vi "Terminal-PressureSystem-DeviceLubricateUnit-Getter.vi"(8 "error in (no error)":errorcluster caption="错误输入（无错误）", 11 "read operation timeout (ms)":i32=5000 caption="读操作超时（5000毫秒）") -> (0 "error out":errorcluster caption="错误输出", 2 "时间标识":timestamp, 3 "液压子系统陪试润滑单元":T1)   [LabVIEW 2014]
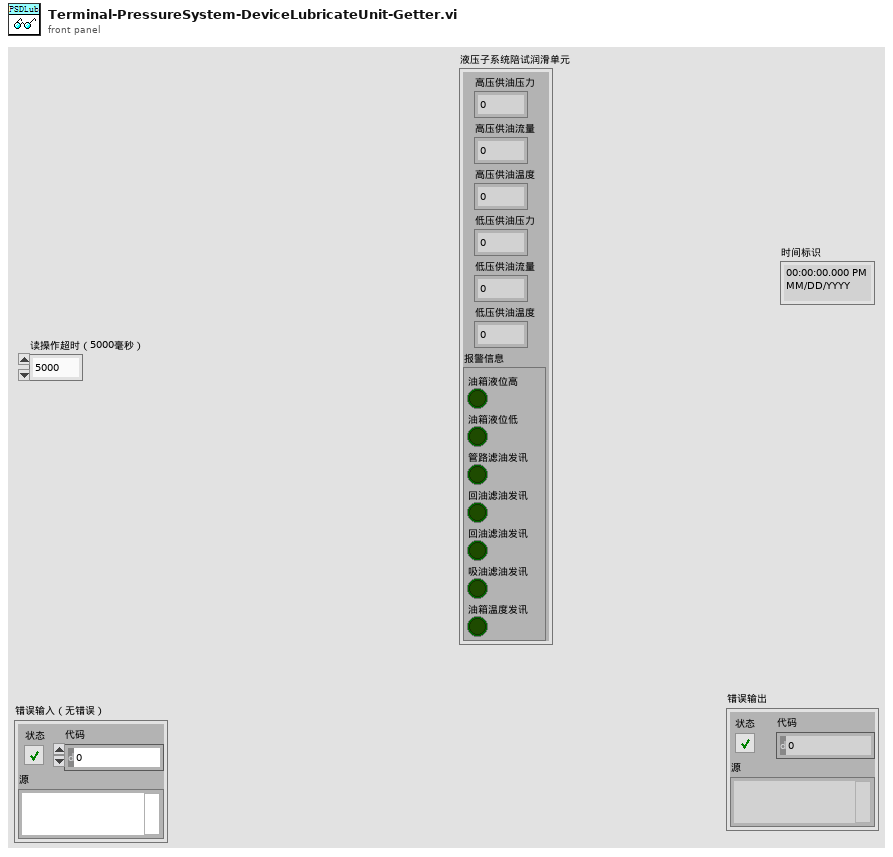
[diagram p1: front panel]
types:
  T1 = cluster{"高压供油压力":u16, "高压供油流量":u16, "高压供油温度":u16, "低压供油压力":u16, "低压供油流量":u16, "低压供油温度":u16, "报警信息":cluster{"油箱液位高":bool, "油箱液位低":bool, "管路滤油发讯":bool, "回油滤油发讯":bool, "回油滤油发讯":bool, "吸油滤油发讯":bool, "油箱温度发讯":bool}}
  T2 = cluster{"油箱液位高":bool, "油箱液位低":bool, "管路滤油发讯":bool, "回油滤油发讯":bool, "回油滤油发讯":bool, "吸油滤油发讯":bool, "油箱温度发讯":bool}
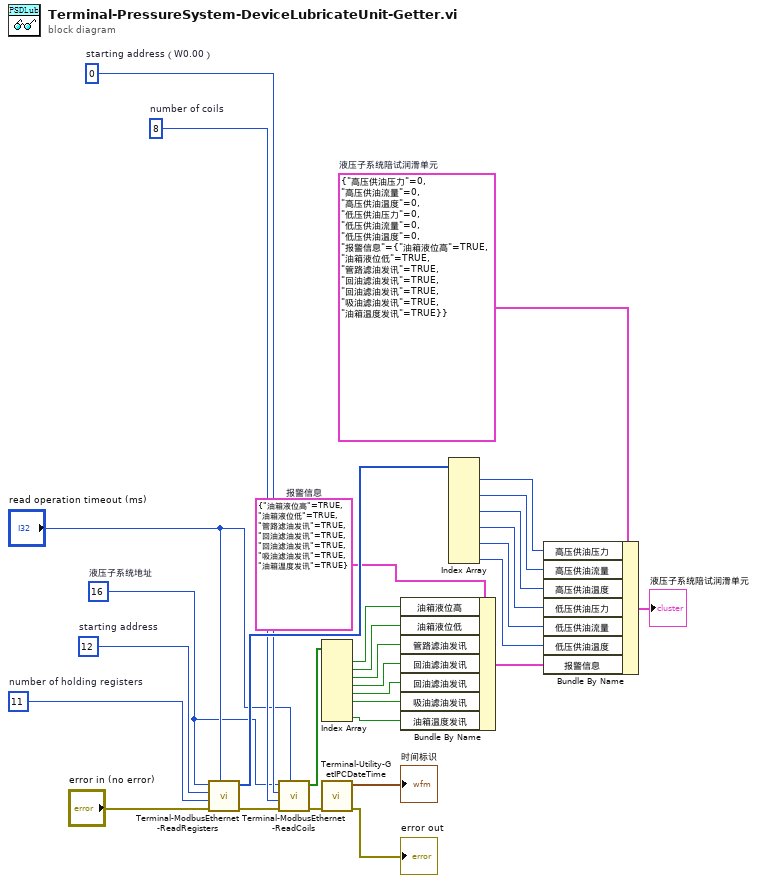
[diagram p0: block diagram]
diagram:
  w12 = T2 {"油箱液位高"=TRUE, "油箱液位低"=TRUE, "管路滤油发讯"=TRUE, "回油滤油发讯"=TRUE, "回油滤油发讯"=TRUE, "吸油滤油发讯"=TRUE, "油箱温度发讯"=TRUE}  # 报警信息
  w21 = u16 8  # number of coils
  w22 = u16 0  # starting address（W0.00）
  w28 = T1 {"高压供油压力"=0, "高压供油流量"=0, "高压供油温度"=0, "低压供油压力"=0, "低压供油流量"=0, "低压供油温度"=0, "报警信息"={"油箱液位高"=TRUE, "油箱液位低"=TRUE, "管路滤油发讯"=TRUE, "回油滤油发讯"=TRUE, "回油滤油发讯"=TRUE, "吸油滤油发讯"=TRUE, "油箱温度发讯"=TRUE}}  # 液压子系统陪试润滑单元
  w7 = u16 11  # number of holding registers
  w30 = u16 12  # starting address
  w8 = u8 16  # 液压子系统地址
  n1 = call "Terminal-ModbusEthernet-ReadRegisters.vi"("read operation timeout (ms)"="read operation timeout (ms)", "error in"="error in (no error)", "number of holding registers"=w7, "starting address"=w30, "unit ID"=w8) -> ("error out"=w1:errorcluster, "register values"=w24:u16[])  [unwired: 5 in]
  n2 = call "Terminal-ModbusEthernet-ReadCoils.vi"("read operation timeout (ms)"="read operation timeout (ms)", "error in"=w1, "number of coils"=w21, "starting address"=w22, "unit ID"=w8) -> ("error out"=w23:errorcluster, "coil values"=w20:bool[])  [unwired: 5 in]
  n3 = Index Array(array=w20) -> (element #1=w19:bool, element #2=w18:bool, element #3=w17:bool, element #4=w16:bool, element #5=w15:bool, element #6=w14:bool, element #8=w10:bool)  [unwired: 8 in, 1 out]
  n4 = call "Terminal-Utility-GetIPCDateTime.vi"("error in (no error)"=w23) -> ("error out"=→"error out":errorcluster, "时间标识"=→"时间标识":timestamp)  [unwired: 9 in]
  n5 = Bundle By Name(cluster=w12, "油箱液位高"=w19, "油箱液位低"=w18, "管路滤油发讯"=w17, "回油滤油发讯"=w16, "回油滤油发讯"=w15, "吸油滤油发讯"=w14, "油箱温度发讯"=w10) -> (w11:T2)
  n6 = Index Array(array=w24) -> (element #1=w27:u16, element #3=w6:u16, element #5=w5:u16, element #7=w4:u16, element #9=w3:u16, element #11=w2:u16)  [unwired: 11 in, 5 out]
  n7 = Bundle By Name(cluster=w28, "高压供油压力"=w27, "高压供油流量"=w6, "高压供油温度"=w5, "低压供油压力"=w4, "低压供油流量"=w3, "低压供油温度"=w2, "报警信息"=w11) -> (→"液压子系统陪试润滑单元":T1)
